vi "Galvo_Reset.vi"(8 "error in":errorcluster, 9 "auto start":bool, 10 "Signal array":dynamicdata[](array[waveform]), 11 "task/channels in":refnum<k21>) -> (0 "error out":errorcluster, 3 "task out":refnum<k21>)   [LabVIEW 2014]
doc: "This SubVI is used to initiate a galvo mirror."
uses:
  <vilib>/DAQmx/write.llb/DAQmx Write (Analog 1D Wfm NChan NSamp).vi
  <vilib>/DAQmx/miscellaneous.llb/DAQmx Fill In Error Info.vi
panel:
  # "This SubVI is used to initiate a galvo mirror."
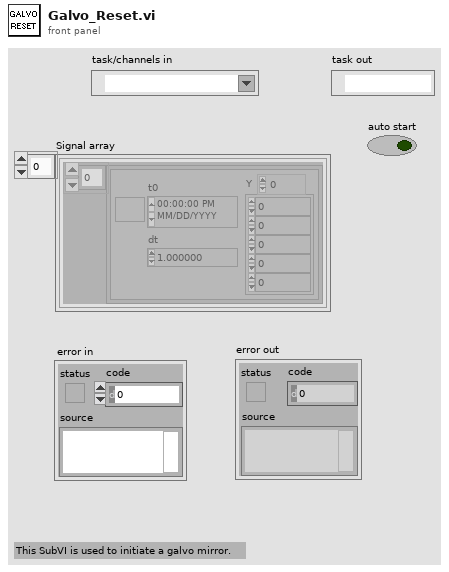
[diagram p1: front panel]
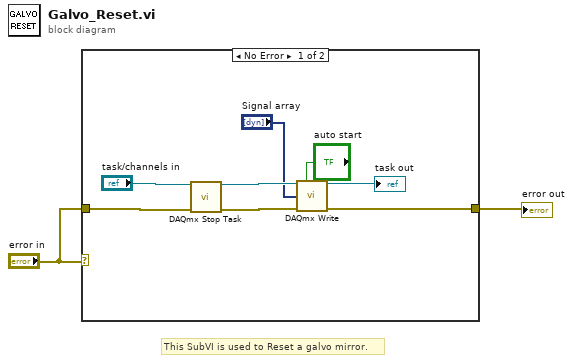
[diagram p0: block diagram]
diagram:
  # "This SubVI is used to Reset a galvo mirror."
  n1 = case shown="No Error" "error in" {
    tunnel: "error in" -> [w10 w11]
    tunnel: [w3 w11] -> w1
    frame No Error {
      n2 = call <vilib>:"DAQmx Stop Task.vi"("task/channels in"="task/channels in", "error in"=w10) -> ("task out"=w8:refnum<k21>, "error out"=w6:errorcluster)  [unwired: 12 in]
      n3 = call-poly <vilib>:"DAQmx Write.vi"("task/channels in"=w8, "auto start"="auto start", "data"="Signal array", "error in"=w6) -> ("task out"=→"task out":refnum<k21>, "error out"=w3:errorcluster)  [unwired: 9 in, 1 out]
    }
    frame Error {
    }
  }
  "error out" <- w1
